vi "Browse Variant_SetRef.vi"(8 "error in (no error)":errorcluster, 10 "Tree Ref":refnum<vi>, 11 "Dummy Class.lvclass in":refnum<class "VariantTree__VP.lvclass">) -> (0 "error out":errorcluster, 3 "Dummy Class.lvclass out":refnum<class "VariantTree__VP.lvclass">)   [LabVIEW 2011, in "VariantTree__VP.lvclass"]
uses:
  VariantTree__VP.lvclass
  VariantTree__VP.lvclass/VariantTree__VP.ctl
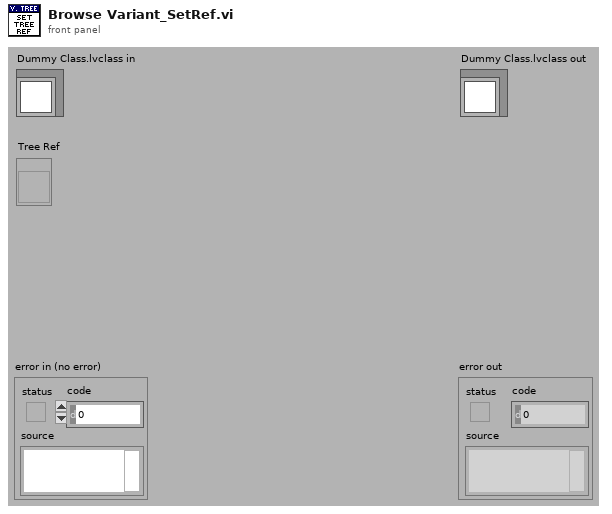
[diagram p1: front panel]
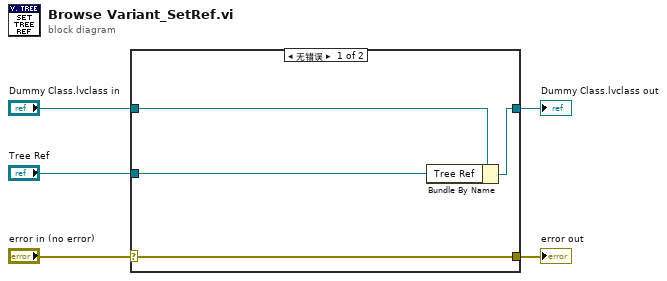
[diagram p0: block diagram]
diagram:
  n1 = case shown="无错误" "error in (no error)" {
    selector: "error in (no error)" -> [w9 w10]
    tunnel: [w9 w10] -> w4
    tunnel: [w7 w11] -> w2
    tunnel: "Dummy Class.lvclass in" -> [w8 w11]
    tunnel: "Tree Ref" -> [w6 _]
    frame No Error {
      n2 = Bundle By Name(cluster=w8, "Tree Ref"=w6) -> (w7:refnum<class "VariantTree__VP.lvclass">)
    }
    frame Error {
    }
  }
  "error out" <- w4
  "Dummy Class.lvclass out" <- w2
